vi "Write pubDataEvents.vi"(10 "pubDataEvents":T1, 11 "Model in":refnum<class "Model.lvclass">) -> (3 "Model out":refnum<class "Model.lvclass">)   [LabVIEW 2013, in "Model.lvclass"]
uses:
  Model.lvclass
  Typedefs/PubDataEvents.ctl
  Typedefs/StateSelector.ctl
  <userlib>/Common/ILC/Typedefs/OutputData.ctl
  <userlib>/Common/ILC/Typedefs/InputData.ctl
  <userlib>/Common/ILC/Configuration/InputChannels.ctl
  <userlib>/Common/ILC/Typedefs/LimitSwitches.ctl
  <userlib>/Common/ILC/Typedefs/ADCs.ctl
  Model.lvclass/Model.ctl
  <userlib>/Common/ILC/Typedefs/ILCTypedefs.lvlib
  <userlib>/Common/ILC/Configuration/ILCConfiguration.lvlib
panel:
  # "DAC"
  # "Limit Switches"
  # "ADCs"
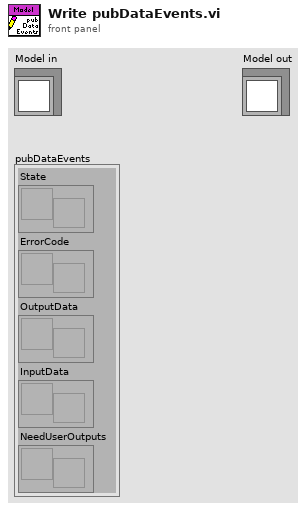
[diagram p1: front panel]
types:
  T1 = typedef "PubDataEvents.ctl" = cluster{"State":refnum<user-event>, "ErrorCode":refnum<user-event>, "OutputData":refnum<user-event>, "InputData":refnum<user-event>, "NeedUserOutputs":refnum<user-event>}
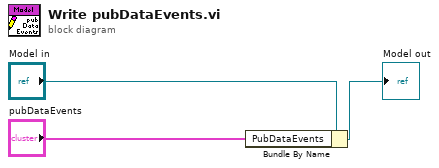
[diagram p0: block diagram]
diagram:
  n1 = Bundle By Name(cluster="Model in", "PubDataEvents"="pubDataEvents") -> (→"Model out":refnum<class "Model.lvclass">)
